vi "Stop.vi"(8 "error in (no error)":errorcluster, 11 "id":i32) -> (0 "error out":errorcluster)   [LabVIEW 2020, in "MCP Server.lvlib"]
doc: "Stops the MCP server."
uses:
  MCP Server.lvlib
  <vilib>/IlluminatedG/IG HTTP Server/HTTP Server/server/Server.lvclass
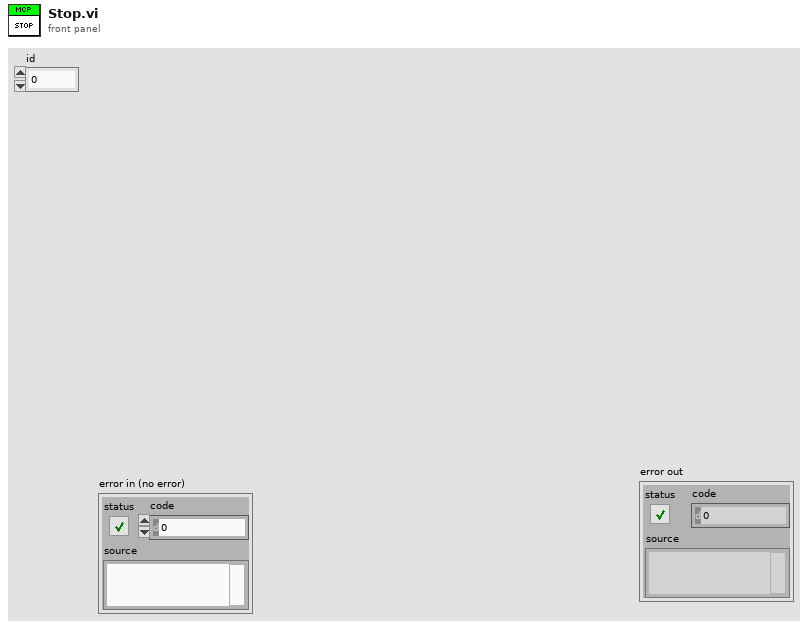
[diagram p1: front panel]
types:
  T1 = enum16{"Get", "GetAll", "Add", "Remove", "Clear"}
  T2 = typedef "MCP Server.lvlib/Server Data.ctl" = cluster{"Name":string, "Description":string, "Tools":T3[], "Parameters":string[][], "Logging Info":T6, "User Events":T7, "Prompts":T8[], "resources":T10[], "HTTP Server":refnum<class "Server.lvclass">}
  T3 = typedef "MCP Server.lvlib/Tool Data.ctl" = cluster{"Name":string, "Description":string, "Ignored":string[], "inputs":T4[], "outputs":T5[], "VI Refnum":refnum<vi>}
  T4 = typedef "MCP Server.lvlib/Input Parameter.ctl" = cluster{"name":string, "type":string, "description":string, "required":bool, "raw name":string}
  T5 = typedef "MCP Server.lvlib/Output Parameter.ctl" = cluster{"name":string, "description":string, "type":string, "raw name":string}
  T6 = typedef "MCP Server.lvlib/Logging.ctl" = cluster{"Log":string[], "Max Length":i32}
  T7 = typedef "MCP Server.lvlib/User Events.ctl" = cluster{"onError":refnum<user-event>, "onRpc":refnum<user-event>}
  T8 = typedef "MCP Server.lvlib/Prompt Data.ctl" = cluster{"name":string, "description":string, "arguments":T9[], "return terminal name":string, "results description":string, "VI Refnum":refnum<vi>}
  T9 = typedef "MCP Server.lvlib/Prompt Argument.ctl" = cluster{"name":string, "description":string, "required":bool, "raw_name":string}
  T10 = typedef "MCP Server.lvlib/resource data.ctl" = cluster{"uri":string, "name":string, "description":string, "mimeType":string, "file path":path}
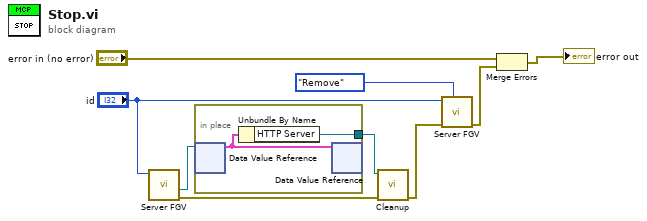
[diagram p0: block diagram]
diagram:
  n1 = call "Server FGV.vi"("id"="id") -> ("error out"=w4:errorcluster, "server reference"=w3:refnum<data-value>)  [unwired: 6 in, 3 out]
  n2 = in-place {
    in-place-border: [w10] -> w2
    n3 = in-place-dvr #1(w3) -> (w11:T2)  [unwired: 1 out]
    n4 = Unbundle By Name(w11) -> ("HTTP Server"=w10:refnum<class "Server.lvclass">)
    n5 = in-place-dvr #1(w11) -> ()  [unwired: 2 out]
  }
  n6 = call <vilib>:"Cleanup.vi"("error in (no error)"=w4, "Server in"=w2) -> ("error out"=w1:errorcluster)  [unwired: 9 in]
  n7 = call "Server FGV.vi"("Mode"=T1."Remove", "error in"=w1, "id"="id") -> ("error out"=w9:errorcluster)  [unwired: 4 in, 4 out]
  n8 = Merge Errors("error in (no error)", w9) -> (→"error out":errorcluster)
